vi "Open Logic VI.vi"(11 "error in":errorcluster) -> (15 "error out":errorcluster)   [LabVIEW 2021, in "Converter.lvlib"]
uses:
  Converter.lvlib
  Path Functions/Path Functions.lvlib
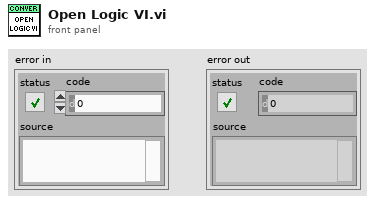
[diagram p1: front panel]
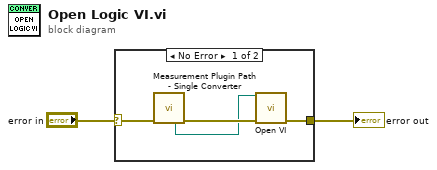
[diagram p0: block diagram]
diagram:
  n1 = case shown="No Error" "error in" {
    selector: "error in" -> [w6 w7]
    tunnel: [w4 w7] -> w1
    frame No Error {
      n2 = call "Measurement Plugin Path - Single Converter.vi"("error in"=w6) -> ("logic vi path"=w3:path, "error out"=w5:errorcluster)  [unwired: 2 in, 11 out]
      n3 = call "Open VI.vi"("logic vi path"=w3, "error in"=w5) -> ("error out"=w4:errorcluster)  [unwired: 13 in]
    }
    frame Error {
    }
  }
  "error out" <- w1
